vi "LcWebView_AlertDialog_Custom General Case.vi"() -> ()   [LabVIEW 2018, in "LcWebView.lvclass"]
uses:
  LcWebView.lvclass
  webui/ctrls/AlertDialogGeneralType.ctl
  webui/ctrls/IconTypeDef.ctl
  C:/Users/ziggz/OneDrive/Documents/GitHub/LcWebView2/LcWebView/LcWebView_class/data/Microsoft.Web.WebView2.WinForms.dll
  data/Microsoft.Web.WebView2.WinForms.dll
panel:
  out "BrowserProcessId":u32
  in  "stop":bool
  out "Result":string
  out "Status Message":string
  in  "Web":refnum<k24>(container)
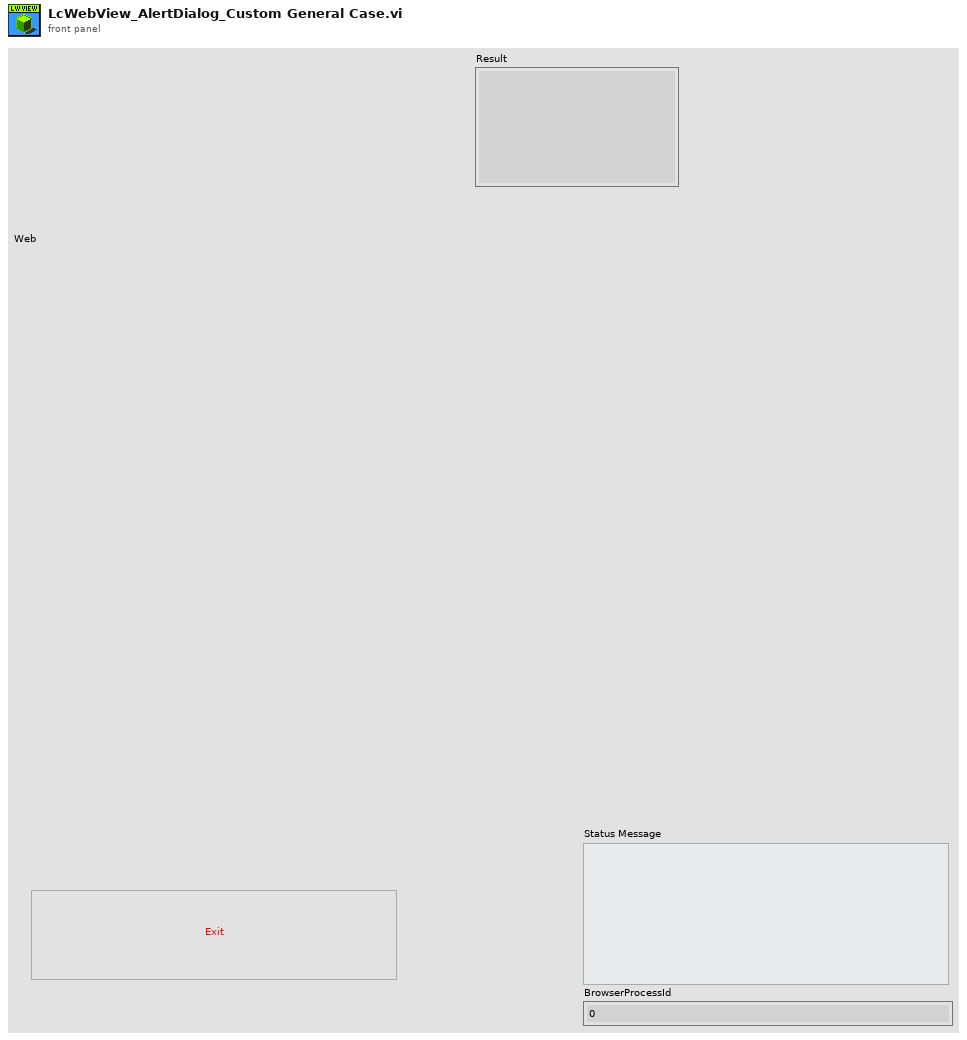
[diagram p1: front panel]
types:
  T1 = typedef "LcWebView.lvclass/AlertDialogGeneralType.ctl" = cluster{"title":string, "titleText":string, "html":string, "text":string, "icon":T2, "iconHtml":string, "showClass":cluster{"popup":string, "backdrop":string, "icon":string}, "hideClass":cluster{"popup":string, "backdrop":string, "icon":string}, "footer":string, "backdrop":bool, "toast":bool, "target":string, "input":string, "width":dbl, "padding":string, "color":string, "background":string, "position":string, "grow":bool, "timer":dbl, "timerProgressBar":bool, "heightAuto":bool, "allowOutsideClick":bool, "allowEscapeKey":bool, "allowEnterKey":bool, "stopKeydownPropagation":bool, "keydownListenerCapture":bool, "showConfirmButton":bool, "showDenyButton":bool, "showCancelButton":bool, "confirmButtonText":string, "denyButtonText":string, "cancelButtonText":string, "confirmButtonColor":string, "denyButtonColor":string, "cancelButtonColor":string, "confirmButtonAriaLabel":string, " denyButtonAriaLabel":string, "cancelButtonAriaLabel":string, "buttonsStyling":bool, "reverseButtons":bool, "focusConfirm":bool, "returnFocus":bool, "focusDeny":bool, "focusCancel":bool}
  T2 = typedef "LcWebView.lvclass/IconTypeDef.ctl" = enum16{"success", "error", "warning", "info", "question"}
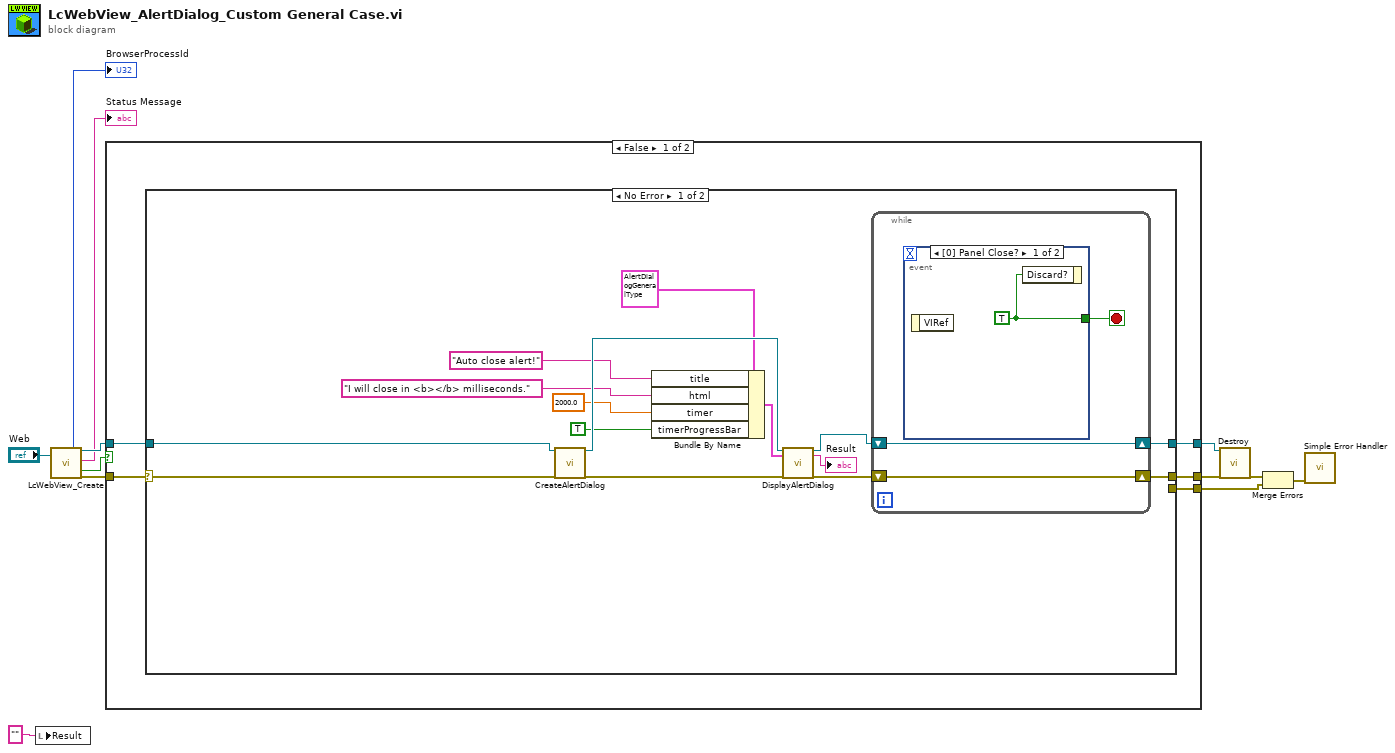
[diagram p0: block diagram]
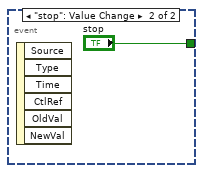
[diagram p2: hidden frame]
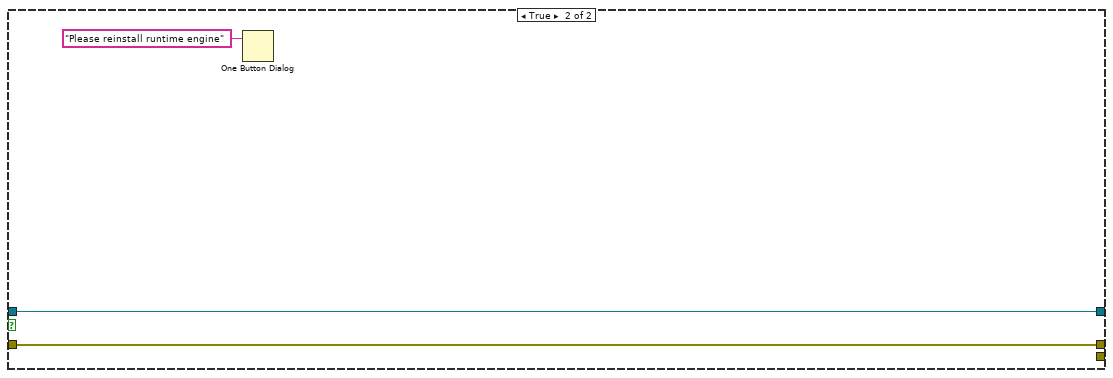
[diagram p4: hidden frame]
diagram:
  n1 = local write "Result"("" ("Result")) -> ()
  n2 = call "LcWebView_Create.vi"("Webview container"="Web") -> ("BrowserProcessId"=→"BrowserProcessId":u32, "reference out"=w11:refnum<class "LcWebView.lvclass">, "Status Message"=→"Status Message":string, "Reinstall Runtime"=w4:bool, "Error Out"=w10:errorcluster)  [unwired: 11 in, 3 out]
  n3 = case shown="False" w4 {
    tunnel: w11 -> [w17 w42]
    tunnel: w10 -> [w16 w41]
    tunnel: [w15 w42] -> w9
    tunnel: [w13 w41] -> w8
    tunnel: [w14 _] -> w5
    frame False {
      n4 = case shown="No Error" w16 {
        selector: w16 -> [w29 w38]
        tunnel: w17 -> [w30 w39]
        tunnel: [w31 w39] -> w15
        tunnel: [w32 _] -> w13
        tunnel: [_ w38] -> w14
        frame No Error {
          n5 = call-dynamic "CreateAlertDialog.vi"("reference in"=w30, "Error In"=w29) -> ("reference out"=w28:refnum<class "LcWebView.lvclass">, "Error Out"=w27:errorcluster)  [unwired: 16 in]
          n6 = Bundle By Name(cluster=T1 {"title"="", "titleText"="", "html"="", "text"="", "icon"=enum."question", "iconHtml"="", "showClass"={"popup"="", "backdrop"="", "icon"=""}, "hideClass"={"popup"="", "backdrop"="", "icon"=""}, "footer"="", "backdrop"=FALSE, "toast"=FALSE, "target"="", "input"="", "width"=0.0, "padding"="", "color"="", "background"="", "position"="", "grow"=FALSE, "timer"=0.0, "timerProgressBar"=FALSE, "heightAuto"=FALSE, "allowOutsideClick"=FALSE, "allowEscapeKey"=FALSE, "allowEnterKey"=FALSE, "stopKeydownPropagation"=FALSE, "keydownListenerCapture"=FALSE, "showConfirmButton"=FALSE, "showDenyButton"=FALSE, "showCancelButton"=FALSE, "confirmButtonText"="", "denyButtonText"="", "cancelButtonText"="", "confirmButtonColor"="", "denyButtonColor"="", "cancelButtonColor"="", "confirmButtonAriaLabel"="", " denyButtonAriaLabel"="", "cancelButtonAriaLabel"="", "buttonsStyling"=FALSE, "reverseButtons"=FALSE, "focusConfirm"=FALSE, "returnFocus"=FALSE, "focusDeny"=FALSE, "focusCancel"=FALSE} ("Alert Dialog Configuration"), "title"="Auto close alert!", "html"="I will close in <b></b> milliseconds.", "timer"=2000.0, "timerProgressBar"=TRUE) -> (w24:T1)
          n7 = call-dynamic "DisplayAlertDialog.vi"("reference in"=w28, "Message"=w24, "Error In"=w27) -> ("reference out"=w26:refnum<class "LcWebView.lvclass">, "Result"=→"Result":string, "Error Out"=w25:errorcluster)  [unwired: 14 in]
          n8 = while {
            shift-right: [w35] -> w31
            shift-left: w26 -> [w35]
            shift-right: [w34] -> w32
            shift-left: w25 -> [w34]
            stop <- w33 stop-if-true
            n9 = event shown="[0] Panel Close?" {
              selector: _ -> [_ _]
              dyn-events: _ -> [_ _]
              timeout: _ -> [_ _]
              tunnel: [w36 "stop"] -> w33
              event Panel Close? {
                w36 = TRUE ("Discard?")
                n10 = event-data() -> ()  [unwired: 1 in, 1 out]
                n11 = event-data("Discard?"=w36) -> ()  [unwired: 1 in, 1 out]
              }
              event "stop": Value Change {
                n12 = event-data() -> ()  [unwired: 1 in, 6 out]
              }
            }
          }
        }
        frame Error {
        }
      }
    }
    frame True {
      n13 = One Button Dialog(message="Please reinstall runtime engine") -> ()  [unwired: 1 in, 1 out]
    }
  }
  n14 = call-dynamic "Destroy.vi"("reference in"=w9, "Error In"=w8) -> ("Error Out"=w7:errorcluster)  [unwired: 16 in, 1 out]
  n15 = Merge Errors(w7, w5) -> (w2:errorcluster)
  n16 = call <vilib>:"Simple Error Handler.vi"("error in (no error)"=w2) -> ()  [unwired: 4 in, 5 out]
